vi "FPGA Calculate X and Y.vi"(9 "Max col":i16, 10 "Row index in":u32, 11 "Current Interation":i32) -> (2 "Col index out":u32, 3 "Row index out":u32)   [LabVIEW 2019]
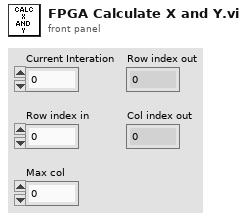
[diagram p1: front panel]
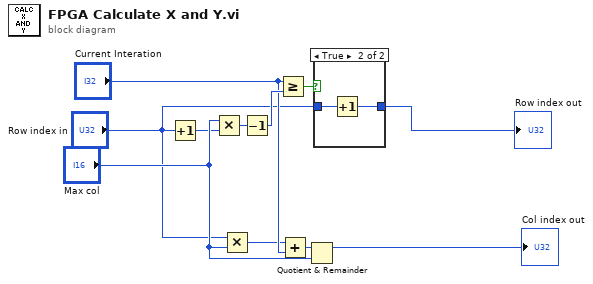
[diagram p0: block diagram]
diagram:
  n1 = Increment(x="Row index in") -> (x+1=w7:u32)
  n2 = Multiply(x="Max col", y=w7) -> (x*y=w1:u32)
  n3 = Multiply(x="Row index in", y="Max col") -> (x*y=w5:u32)
  n4 = Decrement(x=w1) -> (x-1=w8:u32)
  n5 = Greater Or Equal?(x="Current Interation", y=w8) -> (x >= y?=w3:bool)
  n6 = Add(x=w5, y="Current Interation") -> (x+y=w9:u32)
  n7 = Quotient & Remainder(x=w9, y="Max col") -> (x-y*floor(x/y)=→"Col index out":u32)  [unwired: 1 out]
  n8 = case shown="True" w3 {
    tunnel: "Row index in" -> [w12 w14]
    tunnel: [w12 w13] -> w2
    frame False {
    }
    frame True {
      n9 = Increment(x=w14) -> (x+1=w13:u32)
    }
  }
  "Row index out" <- w2
